vi "drive_scaling.vi"(11 "In":dbl) -> (3 "Out":dbl)   [LabVIEW 2013]
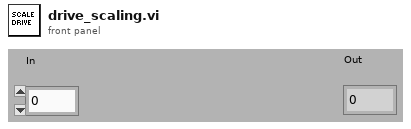
[diagram p1: front panel]
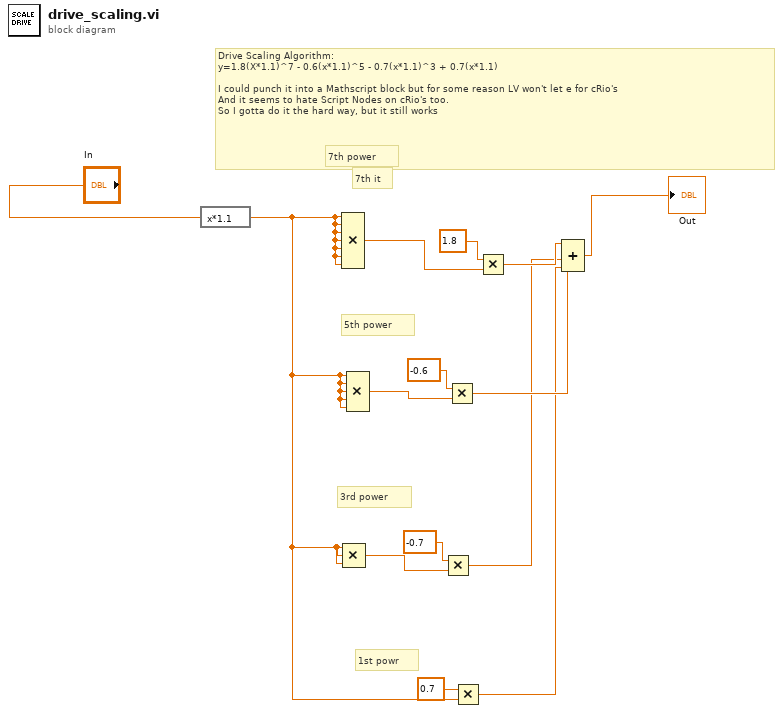
[diagram p0: block diagram]
diagram:
  # "Drive Scaling Algorithm:\ny=1.8(X*1.1)^7 - 0.6(x*1.1)^5 - 0.7(x*1.1)^3 + 0.7(x*1.1)\n\nI could punch it into a Mathscript block but for some reason LV won't let e for cRio's\nAnd it seems to hate Script Nodes on cRio's too.\nSo I gotta do it the hard way, but it still works"
  # "1st powr"
  # "3rd power"
  # "5th power"
  # "7th it"
  # "7th power"
  n1 = expression code="x*1.1"("In") -> (w3:dbl)
  n2 = Compound Arithmetic op=MULTIPLY(w3, w3, w3, w3, w3, w3, w3) -> (w12:dbl)
  n3 = Compound Arithmetic op=MULTIPLY(w3, w3, w3) -> (w5:dbl)
  n4 = Compound Arithmetic op=MULTIPLY(w3, w3, w3, w3, w3) -> (w8:dbl)
  n5 = Multiply(x=-0.7, y=w5) -> (x*y=w4:dbl)
  n6 = Multiply(x=-0.6, y=w8) -> (x*y=w7:dbl)
  n7 = Multiply(x=0.7, y=w3) -> (x*y=w1:dbl)
  n8 = Multiply(x=1.8, y=w12) -> (x*y=w11:dbl)
  n9 = Compound Arithmetic op=ADD(w11, w7, w4, w1) -> (→"Out":dbl)
